vi "Robot Global Data V.3.0.vi"() -> ()   [LabVIEW 2017]
doc: "This global VI can contain as many global variables as you need. Place a control on the panel, give it a good name. To read or write to it from a VI, drag the icon to the diagram of that VI. You can also drag from the project. Click on the node to change which global you access. You shouldn't have multiple locations writing to a global or it will cause a race-condition."
uses:
  <vilib>/Rock Robotics/WPI/Camera/WPI_CameraImageSize.ctl
  <vilib>/Rock Robotics/WPI/DriverStation/WPI_DriverStationRobotMode2.ctl
panel:
  in  "Automatic Arms Up and Scale Angle":bool
  in  "Right Encoder Initial":dbl
  in  "Left Encoder Intial":dbl
  in  "Atlas?":bool
  in  "Automatic Arms Down and Collector In":bool
  in  "Fast Drive Mode":bool
  in  "Slow Drive Mode":bool
  in  "Kicker Drive Latch":bool
  in  "Intake Hold":bool
  in  "Bring Collector Fully Out?":bool
  in  "Bring Collector Fully In?":bool
  in  "Gyro":dbl
  in  "Kicker Latch":bool
  in  "Right Dart Amps":dbl
  in  "Left Dart Amps":dbl
  in  "Collector Speed":dbl
  in  "Left Dart Final Speed":dbl
  in  "Right Dart Final Speed":dbl
  in  "Right Collector Intake Motor Speed":dbl
  in  "Left Collector Intake Motor Speed":dbl
  in  "Right Collector Intake Motor Amps":dbl
  in  "Left Collector Intake Motor Amps":dbl
  in  "Collector Angle Motor Actual Angle":dbl
  in  "Collector Angle Motor Wanted Angle":dbl
  in  "# of the Right Dart":i32
  in  "# of the Left Dart":i32
  in  "Dart #4":T1
  in  "Dart #3":T1
  in  "Dart #2":T1
  in  "Dart #1":T1
  in  "Collector Latch":bool
  in  "Shoot Cube":bool
  in  "Right Dart Speed Before Fix":dbl
  in  "Left Dart Speed Before Fix":dbl
  in  "Right Dart Fix":dbl
  in  "Left Dart Fix":dbl
  in  "Tank?":bool
  in  "Drive Speed Fix":dbl
  in  "Right Potentiometer Actual Value":dbl
  in  "Left Aux Joystick Y":dbl
  in  "Left Aux Joystick X":dbl
  in  "Right Aux Joystick Y":dbl
  in  "Right Aux Joystick X":dbl
  in  "Left Potentiometer Actual Value":dbl
  in  "Encoder Right":dbl
  in  "Encoder Left":dbl
  in  "Left Drive Joystick Y":dbl
  in  "Left Drive Joystick X":dbl
  in  "Right Drive Joystick Y":dbl
  in  "Right Drive Joystick X":dbl
  in  "Robot Mode":T2
  in  "image size":T3=enum."320x240"
  in  "Enable Vision":bool
  # "Joystick"
  # "Sensors"
  # "if you would like to change the tables, change\nin robot main.vi where they are hard-coded"
  # "if you would like to change, change\nin begin.vi where they are hard-coded"
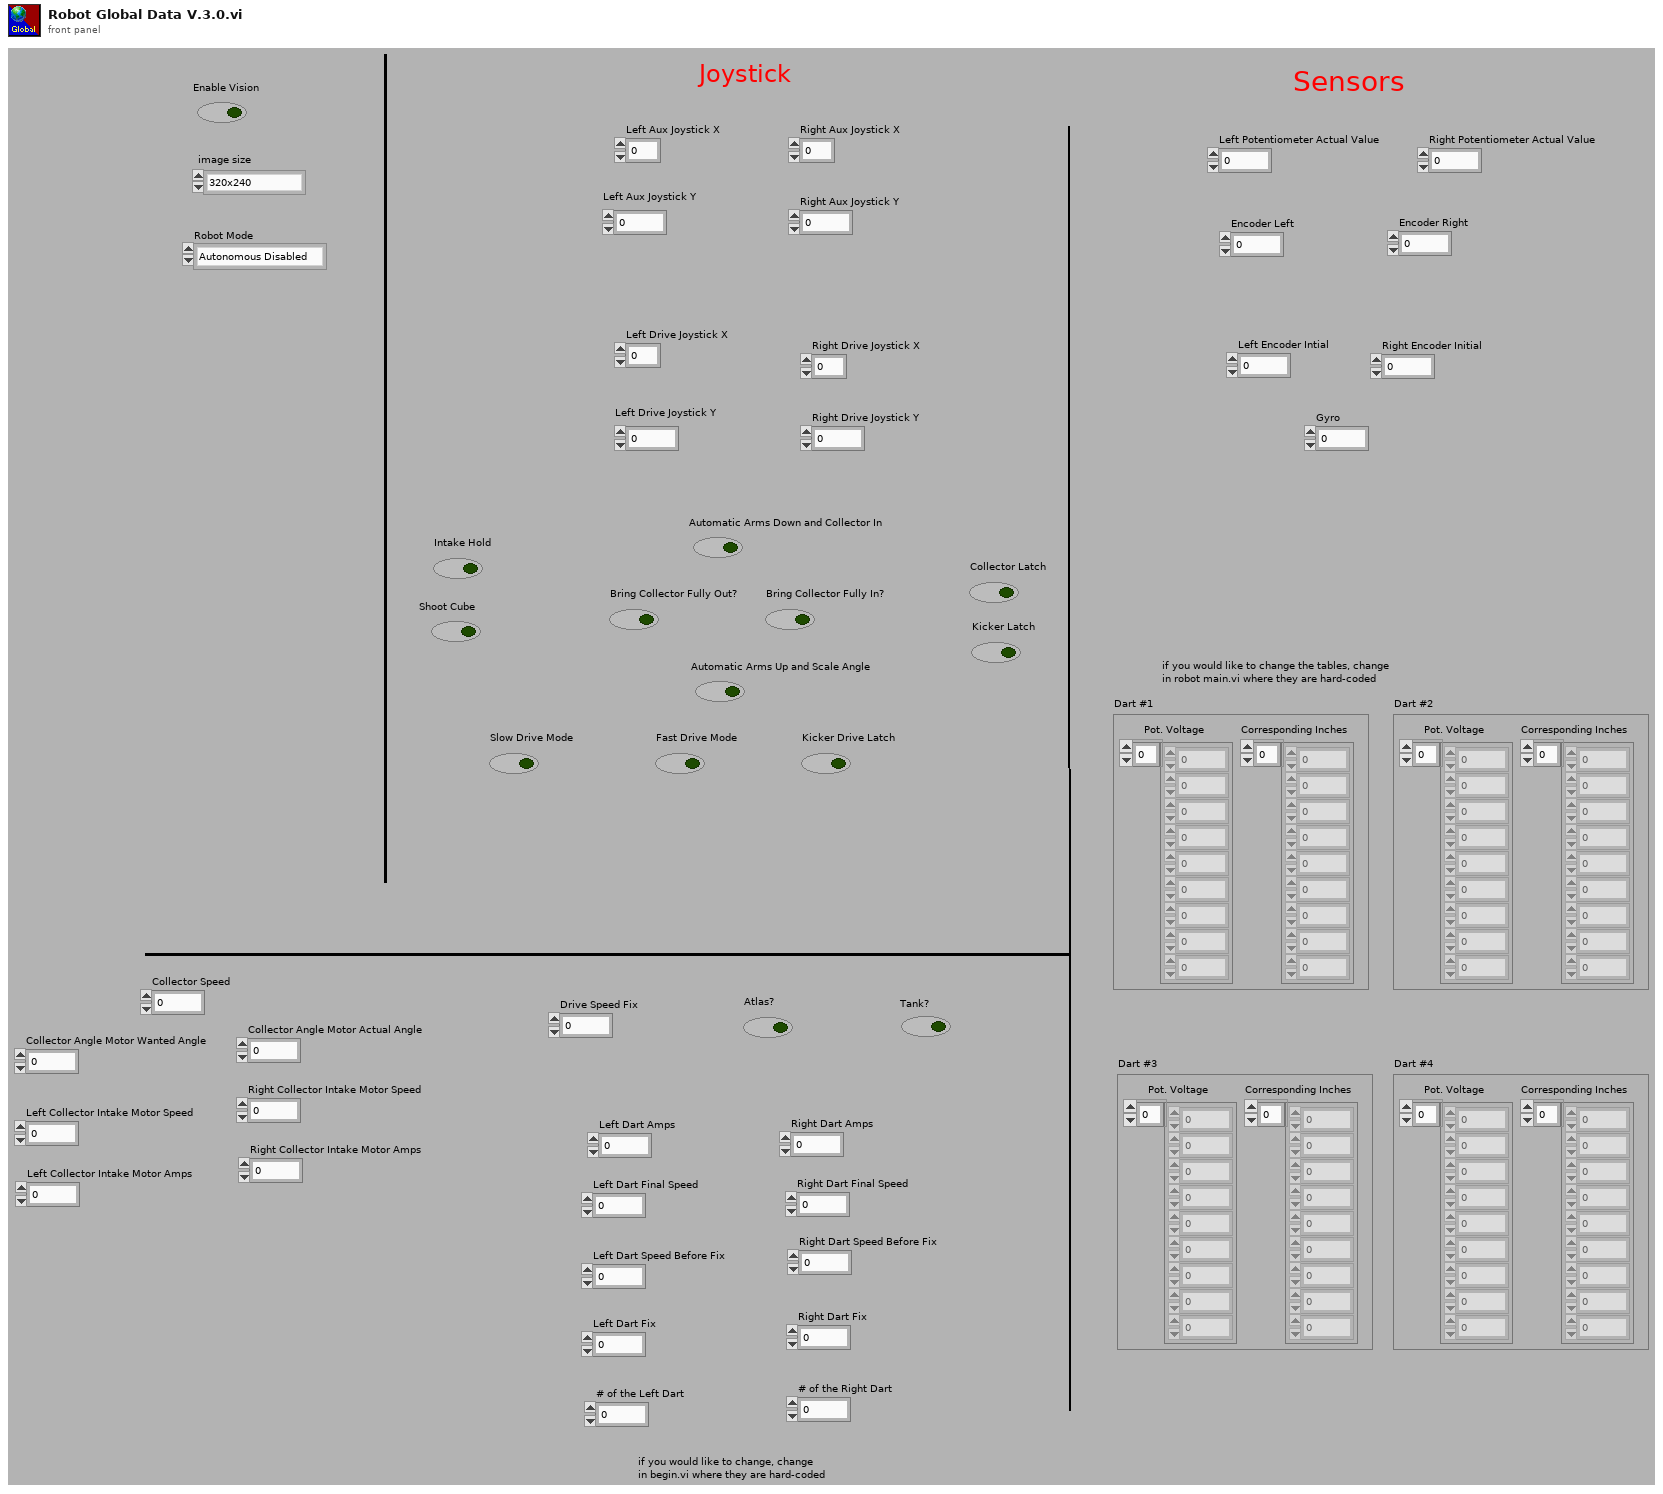
[diagram p1: front panel]
types:
  T1 = cluster{"Pot. Voltage":dbl[], "Corresponding Inches":dbl[]}
  T2 = typedef "WPI_DriverStationRobotMode2.ctl" = enum16{"Autonomous Disabled", "Autonomous Enabled", "Teleop Disabled", "Teleop Enabled", "Disconnected", "Finish", "Test Disabled", "Test Enabled", "Emergency Stopped"}
  T3 = typedef "WPI_CameraImageSize.ctl" = enum16{"640x480", "320x240", "160x120", "Custom"}
diagram:
